vi "B_WriteProperty.vi"(8 "Error In":errorcluster, 10 "Property":dbl, 11 "reference in":refnum<class "BaseTemplate_4x4x4.lvclass">) -> (0 "Error Out":errorcluster, 3 "reference out":refnum<class "BaseTemplate_4x4x4.lvclass">)   [LabVIEW 2020]
uses:
  <resource>/Framework/Providers/Open_GDS/ClassProviders/Provider_EndevoGOOP300/Templates/BaseTemplate_4x4x4/BaseTemplate_4x4x4.lvclass
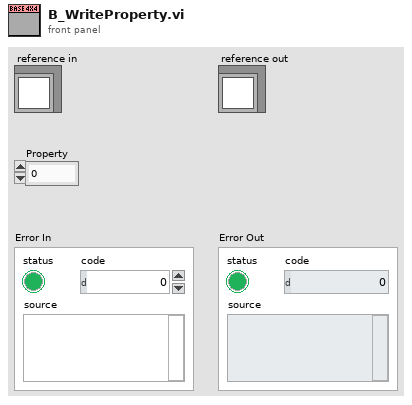
[diagram p1: front panel]
types:
  T1 = typedef "BaseTemplate_4x4x4.lvclass/ObjectAttributes.ctl" = cluster{"Attribute1":dbl}
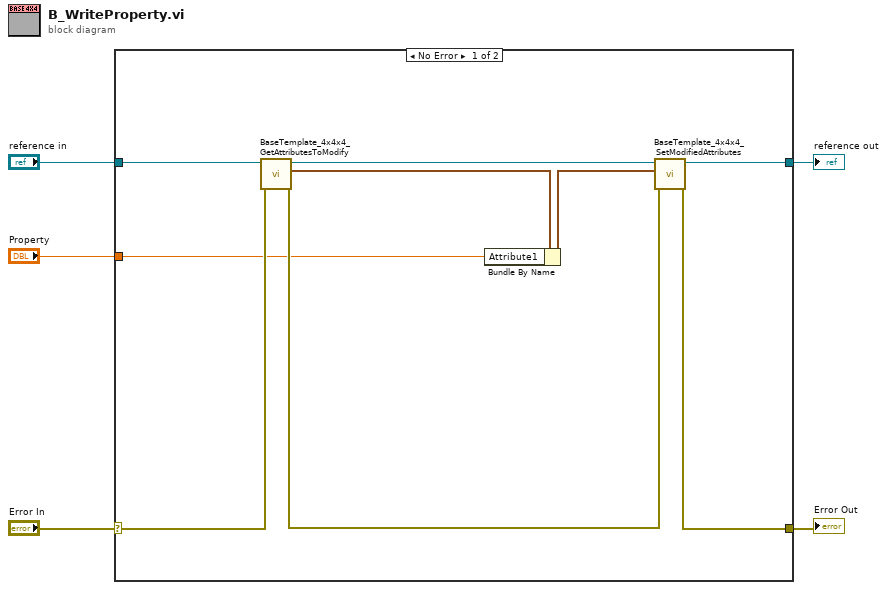
[diagram p0: block diagram]
diagram:
  n1 = case shown="No Error" "Error In" {
    selector: "Error In" -> [w9 w16]
    tunnel: [w11 w16] -> w4
    tunnel: [w8 w15] -> w2
    tunnel: "reference in" -> [w10 w15]
    tunnel: "Property" -> [w6 _]
    frame No Error {
      n2 = call <resource>:"BaseTemplate_4x4x4_GetAttributesToModify.vi"("error in (no error)"=w9, "reference in"=w10) -> ("error out"=w7:errorcluster, "Attributes"=w14:T1, "reference out"=w12:refnum<class "BaseTemplate_4x4x4.lvclass">)  [unwired: 6 in, 1 out]
      n3 = Bundle By Name(cluster=w14, "Attribute1"=w6) -> (w13:T1)
      n4 = call <resource>:"BaseTemplate_4x4x4_SetModifiedAttributes.vi"("error in (no error)"=w7, "Attributes"=w13, "reference in"=w12) -> ("error out"=w11:errorcluster, "reference out"=w8:refnum<class "BaseTemplate_4x4x4.lvclass">)  [unwired: 7 in]
    }
    frame Error {
    }
  }
  "Error Out" <- w4
  "reference out" <- w2
